vi "MNIST_Read_Dataset(In1D_Out1D).vi"(7 "MNIST Dataset Path":path=path "D:/DNN/data/DataSets/MNIST/train-images.idx3-ubyte", 8 "error in":errorcluster, 10 "Validation_Size":sgl=0.1) -> (0 "error out":errorcluster, 3 "Datasets(Train,Val,Test)":T1={"Train"={"Inputs Ref."=variant(refnum<data-value> refnum), "Outputs Ref."=refnum, "Dims_In"=784, "Dataset_Size"=59000, "Dims_Out"=0, "Labels"=[], "File Paths"=[]}, "Validation"={"Inputs Ref."=variant(refnum<data-value> refnum), "Outputs Ref."=refnum, "Dims_In"=784, "Dataset_Size"=1000, "Dims_Out"=0, "Labels"=[], "File Paths"=[]}, "Test"={"Inputs Ref."=variant(refnum<data-value> refnum), "Outputs Ref."=refnum, "Dims_In"=784, "Dataset_Size"=10000, "Dims_Out"=0, "Labels"=[], "File Paths"=[]}})   [LabVIEW 2020]
uses:
  <vilib>/Ngene/Deep Learning Toolkit/Toolkit/NN_Data/API/DataSet/DataSet_Types/NN_DataSets_All(In1D_Out1D).ctl
  <vilib>/Ngene/Deep Learning Toolkit/Toolkit/NN_Data/API/DataSet/DataSet_Types/NN_DataSet(In1D_Out1D).ctl
  <vilib>/Ngene/Deep Learning Toolkit/Toolkit/NN_Data/Controls/DataRef_Types/2D/NN_Data_ref(2D_SGL).ctl
  <vilib>/Ngene/Deep Learning Toolkit/Toolkit/NN_Data/subVIs/Dataset_Split/NN_DataSet_Split(In1D_Out1D).vi
  <vilib>/Ngene/Deep Learning Toolkit/Toolkit/Deep_Learning_Toolkit_by_Ngene.lvlib
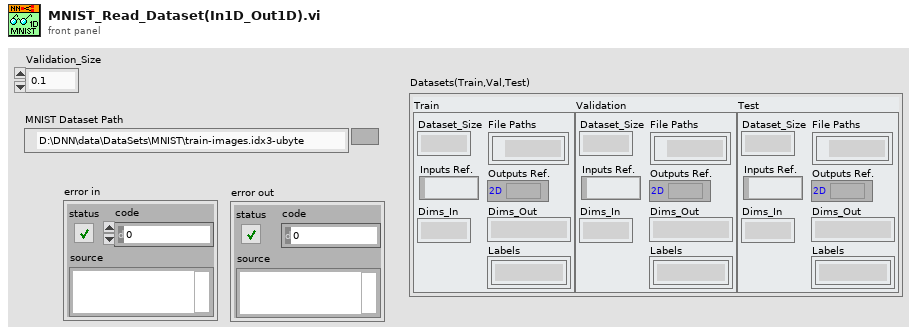
[diagram p1: front panel]
types:
  T1 = typedef "Deep_Learning_Toolkit_by_Ngene.lvlib/NN_DataSets_All(In1D_Out1D).ctl" = cluster{"Train":T2, "Validation":T2, "Test":T2}
  T2 = typedef "Deep_Learning_Toolkit_by_Ngene.lvlib/NN_DataSet(In1D_Out1D).ctl" = cluster{"Inputs Ref.":variant, "Outputs Ref.":T3, "Dims_In":i32, "Dataset_Size":i32, "Dims_Out":i32, "Labels":string[], "File Paths":path[]}
  T3 = typedef "Deep_Learning_Toolkit_by_Ngene.lvlib/NN_Data_ref(2D_SGL).ctl" = refnum<data-value>
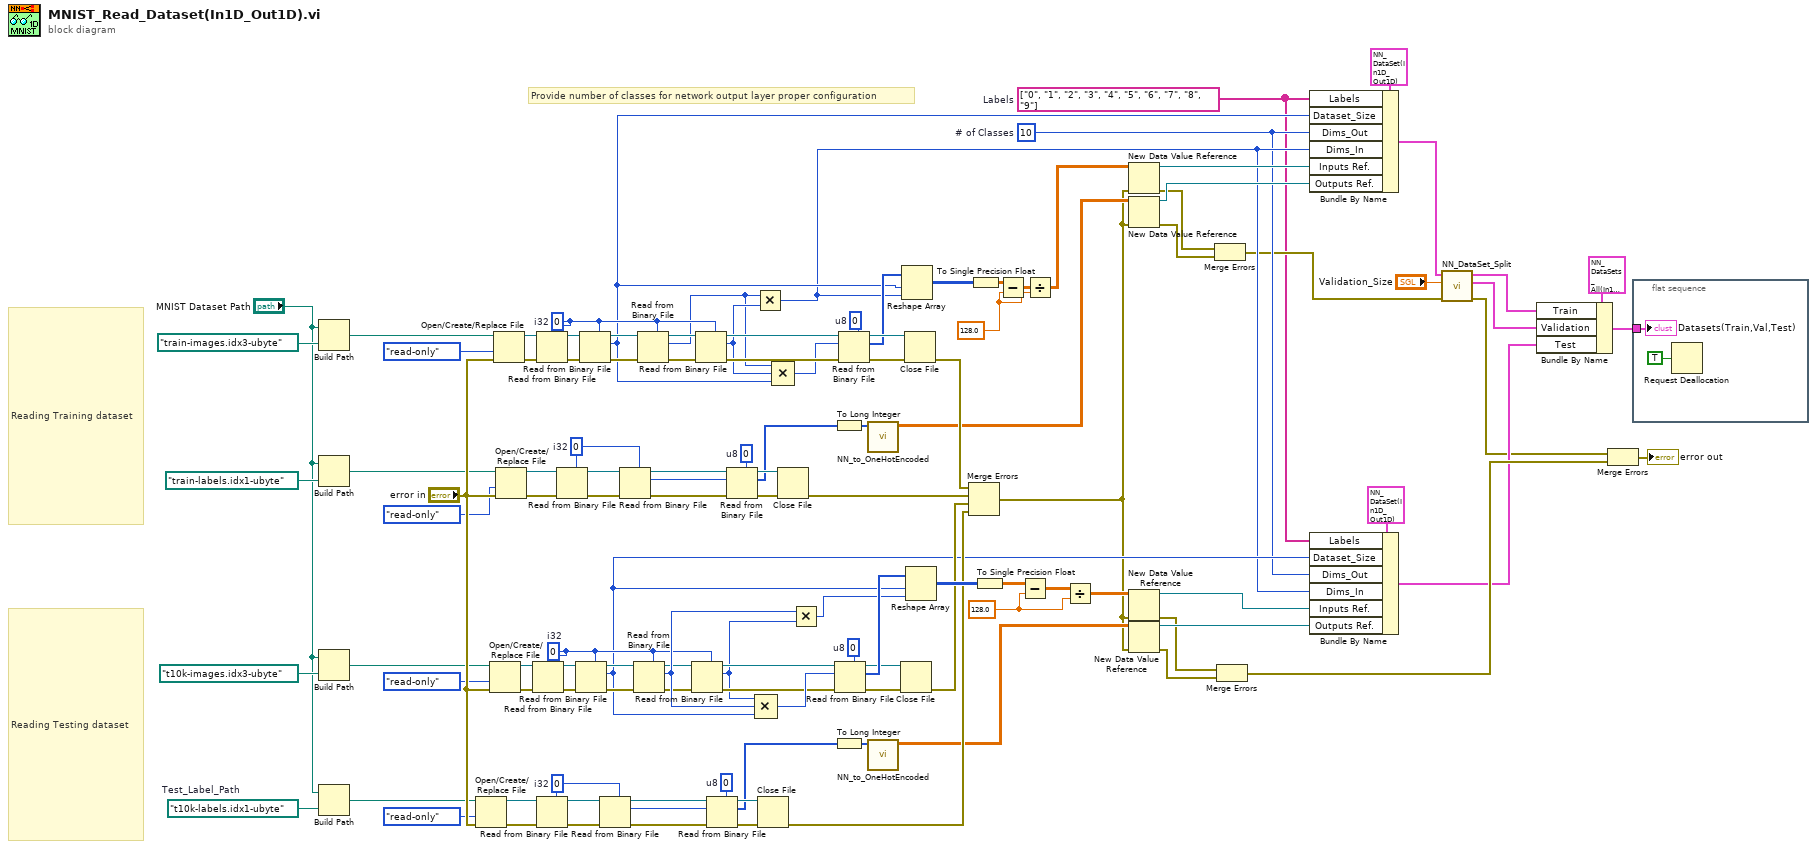
[diagram p0: block diagram]
diagram:
  w6 = string[] ["0", "1", "2", "3", "4", "5", "6", "7", "8", "9"]  # Labels
  w13 = 10  # # of Classes
  w26 = path "t10k-labels.idx1-ubyte"  # Test_Label_Path
  w14 = sgl 128.0 ("y")
  w16 = sgl 128.0 ("y")
  w88 = u8 0  # u8
  w87 = u8 0  # u8
  w79 = 0  # i32
  w68 = 0  # i32
  w94 = u8 0  # u8
  w95 = u8 0  # u8
  w103 = 0  # i32
  w115 = 0  # i32
  # "Provide number of classes for network output layer proper configuration"
  # "Reading Testing dataset"
  # "Reading Training dataset"
  n1 = Build Path(base path="MNIST Dataset Path", name or relative path=path "train-images.idx3-ubyte" ("Train_Image_Path")) -> (appended path=w23:path)
  n2 = Build Path(base path="MNIST Dataset Path", name or relative path=path "train-labels.idx1-ubyte" ("Train_Label_Path")) -> (appended path=w22:path)
  n3 = Build Path(base path="MNIST Dataset Path", name or relative path=path "t10k-images.idx3-ubyte" ("Test_Image_Path")) -> (appended path=w21:path)
  n4 = Build Path(base path="MNIST Dataset Path", name or relative path=w26) -> (appended path=w20:path)
  n5 = Open/Create/Replace File(file path (use dialog)=w20, error in="error in", access (0:read/write)=enum16{"read/write", "read-only", "write-only"}."read-only") -> (refnum out=w81:refnum<file>, error out=w78:errorcluster)  [unwired: 3 in, 1 out]
  n6 = Open/Create/Replace File(file path (use dialog)=w21, error in="error in", access (0:read/write)=enum16{"read/write", "read-only", "write-only"}."read-only") -> (refnum out=w64:refnum<file>, error out=w70:errorcluster)  [unwired: 3 in, 1 out]
  n7 = Open/Create/Replace File(file path (use dialog)=w23, error in="error in", access (0:read/write)=enum16{"read/write", "read-only", "write-only"}."read-only") -> (refnum out=w119:refnum<file>, error out=w113:errorcluster)  [unwired: 3 in, 1 out]
  n8 = Open/Create/Replace File(file path (use dialog)=w22, error in="error in", access (0:read/write)=enum16{"read/write", "read-only", "write-only"}."read-only") -> (refnum out=w101:refnum<file>, error out=w104:errorcluster)  [unwired: 3 in, 1 out]
  n9 = Read from Binary File(5:w68, 8:w70, 11:w64) -> (0:w71:errorcluster, 3:w65:refnum<file>)  [unwired: 3 in, 2 out]
  n10 = Read from Binary File(5:w115, 8:w113, 11:w119) -> (0:w112:errorcluster, 3:w118:refnum<file>)  [unwired: 3 in, 2 out]
  n11 = Read from Binary File(5:w79, 8:w78, 11:w81) -> (0:w77:errorcluster, 3:w80:refnum<file>)  [unwired: 3 in, 2 out]
  n12 = Read from Binary File(5:w103, 8:w104, 11:w101) -> (0:w105:errorcluster, 3:w102:refnum<file>)  [unwired: 3 in, 2 out]
  n13 = Read from Binary File(5:w68, 8:w71, 11:w65) -> (0:w72:errorcluster, 2:w42:i32, 3:w67:refnum<file>)  [unwired: 3 in, 1 out]
  n14 = Read from Binary File(5:w115, 8:w112, 11:w118) -> (0:w111:errorcluster, 2:w19:i32, 3:w116:refnum<file>)  [unwired: 3 in, 1 out]
  n15 = Read from Binary File(5:w79, 8:w77, 11:w80) -> (0:w83:errorcluster, 2:w35:i32, 3:w82:refnum<file>)  [unwired: 3 in, 1 out]
  n16 = Read from Binary File(5:w103, 8:w105, 11:w102) -> (0:w99:errorcluster, 2:w36:i32, 3:w100:refnum<file>)  [unwired: 3 in, 1 out]
  n17 = Read from Binary File(5:w68, 8:w72, 11:w67) -> (0:w73:errorcluster, 2:w89:i32, 3:w66:refnum<file>)  [unwired: 3 in, 1 out]
  n18 = Read from Binary File(5:w115, 8:w111, 11:w116) -> (0:w110:errorcluster, 2:w93:i32, 3:w117:refnum<file>)  [unwired: 3 in, 1 out]
  n19 = Read from Binary File(5:w68, 8:w73, 11:w66) -> (0:w74:errorcluster, 2:w41:i32, 3:w69:refnum<file>)  [unwired: 3 in, 1 out]
  n20 = Read from Binary File(5:w115, 8:w110, 11:w117) -> (0:w109:errorcluster, 2:w107:i32, 3:w114:refnum<file>)  [unwired: 3 in, 1 out]
  n21 = Read from Binary File(5:w88, 8:w83, 10:w35, 11:w82) -> (0:w85:errorcluster, 2:w34:u8[], 3:w84:refnum<file>)  [unwired: 2 in, 1 out]
  n22 = Read from Binary File(5:w94, 8:w99, 10:w36, 11:w100) -> (0:w97:errorcluster, 2:w91:u8[], 3:w98:refnum<file>)  [unwired: 2 in, 1 out]
  n23 = Multiply(x=w93, y=w107) -> (x*y=w18:i32)
  n24 = Compound Arithmetic op=MULTIPLY(w41, w89, w42) -> (w76:i32)
  n25 = Close File(refnum=w84, error in=w85) -> (error out=w51:errorcluster)  [unwired: 1 out]
  n26 = Compound Arithmetic op=MULTIPLY(w93, w107, w19) -> (w106:i32)
  n27 = Close File(refnum=w98, error in=w97) -> (error out=w53:errorcluster)  [unwired: 1 out]
  n28 = Multiply(x=w89, y=w41) -> (x*y=w43:i32)
  n29 = To Long Integer(number=w91) -> (32bit integer=w5:i32[])
  n30 = To Long Integer(number=w34) -> (32bit integer=w3:i32[])
  n31 = Read from Binary File(5:w87, 8:w74, 10:w76, 11:w69) -> (0:w75:errorcluster, 2:w86:u8[], 3:w63:refnum<file>)  [unwired: 2 in, 1 out]
  n32 = Read from Binary File(5:w95, 8:w109, 10:w106, 11:w114) -> (0:w108:errorcluster, 2:w96:u8[], 3:w120:refnum<file>)  [unwired: 2 in, 1 out]
  n33 = call <vilib>:"NN_to_OneHotEncoded.vi"("Label_Idx"=w5) -> ("Prediction"=w4:sgl[][])  [unwired: 10 in]
  n34 = call <vilib>:"NN_to_OneHotEncoded.vi"("Label_Idx"=w3) -> ("Prediction"=w2:sgl[][])  [unwired: 10 in]
  n35 = Close File(refnum=w63, error in=w75) -> (error out=w52:errorcluster)  [unwired: 1 out]
  n36 = Reshape Array(w96, w19, w18) -> (w92:u8[][])
  n37 = Close File(refnum=w120, error in=w108) -> (error out=w54:errorcluster)  [unwired: 1 out]
  n38 = Reshape Array(w86, w42, w43) -> (w90:u8[][])
  n39 = Merge Errors(w54, w53, w52, w51) -> (w1:errorcluster)
  n40 = To Single Precision Float(number=w92) -> (single precision float=w55:sgl[][])
  n41 = To Single Precision Float(number=w90) -> (single precision float=w56:sgl[][])
  n42 = Subtract(x=w55, y=w16) -> (x-y=w29:sgl[][])
  n43 = Subtract(x=w56, y=w14) -> (x-y=w30:sgl[][])
  n44 = Divide(x=w29, y=w16) -> (x/y=w17:sgl[][])
  n45 = Divide(x=w30, y=w14) -> (x/y=w15:sgl[][])
  n46 = New Data Value Reference(data value=w17, error in=w1) -> (data value reference=w61:refnum<data-value>, error out=w49:errorcluster)
  n47 = New Data Value Reference(data value=w4, error in=w1) -> (data value reference=w60:refnum<data-value>, error out=w50:errorcluster)
  n48 = New Data Value Reference(data value=w15, error in=w1) -> (data value reference=w58:refnum<data-value>, error out=w48:errorcluster)
  n49 = New Data Value Reference(data value=w2, error in=w1) -> (data value reference=w59:refnum<data-value>, error out=w47:errorcluster)
  n50 = Merge Errors(w49, w50) -> (w8:errorcluster)
  n51 = Merge Errors(w48, w47) -> (w46:errorcluster)
  n52 = Bundle By Name(cluster=T2 {"Inputs Ref."=variant(refnum<data-value> refnum), "Outputs Ref."=refnum, "Dims_In"=0, "Dataset_Size"=0, "Dims_Out"=0, "Labels"=[], "File Paths"=[]} ("Test_Data"), "Labels"=w6, "Dataset_Size"=w19, "Dims_Out"=w13, "Dims_In"=w18, "Inputs Ref."=w61, "Outputs Ref."=w60) -> (w12:T2)
  n53 = Bundle By Name(cluster=T2 {"Inputs Ref."=variant(refnum<data-value> refnum), "Outputs Ref."=refnum, "Dims_In"=0, "Dataset_Size"=0, "Dims_Out"=0, "Labels"=[], "File Paths"=[]} ("Test_Data"), "Labels"=w6, "Dataset_Size"=w42, "Dims_Out"=w13, "Dims_In"=w18, "Inputs Ref."=w58, "Outputs Ref."=w59) -> (w33:T2)
  n54 = call-poly <vilib>:"NN_DataSet_Split.vi"("error in(no error)"=w8, "Split Size"="Validation_Size", "Dataset In"=w12) -> ("error out"=w7:errorcluster, "Dataset Out 2"=w9:T2, "Dataset Out 1"=w10:T2)  [unwired: 6 in]
  n55 = Bundle By Name(cluster=T1 {"Train"={"Inputs Ref."=variant(refnum<data-value> refnum), "Outputs Ref."=refnum, "Dims_In"=0, "Dataset_Size"=0, "Dims_Out"=0, "Labels"=[], "File Paths"=[]}, "Validation"={"Inputs Ref."=variant(refnum<data-value> refnum), "Outputs Ref."=refnum, "Dims_In"=0, "Dataset_Size"=0, "Dims_Out"=0, "Labels"=[], "File Paths"=[]}, "Test"={"Inputs Ref."=variant(refnum<data-value> refnum), "Outputs Ref."=refnum, "Dims_In"=0, "Dataset_Size"=0, "Dims_Out"=0, "Labels"=[], "File Paths"=[]}} ("Data_Refs"), "Train"=w10, "Validation"=w9, "Test"=w33) -> (w32:T1)
  n56 = Merge Errors(w7, w46) -> (→"error out":errorcluster)
  n57 = flat-sequence {
    tunnel: w32 -> [w121]
    frame #0 {
      n58 = Request Deallocation(TRUE ("flag")) -> ()
      "Datasets(Train,Val,Test)" <- w121
    }
  }
